vi "Pass Fail and Report Text.vi"(0 "Previous Fault Count":u8, 2 "Mode":T1, 5 "Faults Cleared":T2[](array[typedef]) {"ERD Number" format="%.0x"}, 7 "Faults Active":T2[](array[typedef]) {"ERD Number" format="%.0x"}, 9 "Motor Stopped":T2[][](array[typedef]) {"ERD Number" format="%.0x"}, 11 "Error In":errorcluster, 13 "Motor Running":T2[][](array[typedef]) {"ERD Number" format="%.0x"}) -> (4 "Pass/Fail?":bool, 6 "Report Text":string, 8 "Current Fault Count":u8, 15 "Error Out":errorcluster)   [LabVIEW 2016, in "Centauro.lvlib"]
doc: "This VI generates pass/fail and report text data based on the output of the locked rotor test VI."
uses:
  Projects/Centauro.lvlib
  Common/LabVIEW GEA2 Toolkit/LabVIEW_GEA2_Toolkit.lvlibp/type defs/ERD Read Data Out.ctl
  controls/Mode.ctl
  Common/LabVIEW GEA2 Toolkit/LabVIEW_GEA2_Toolkit.lvlibp
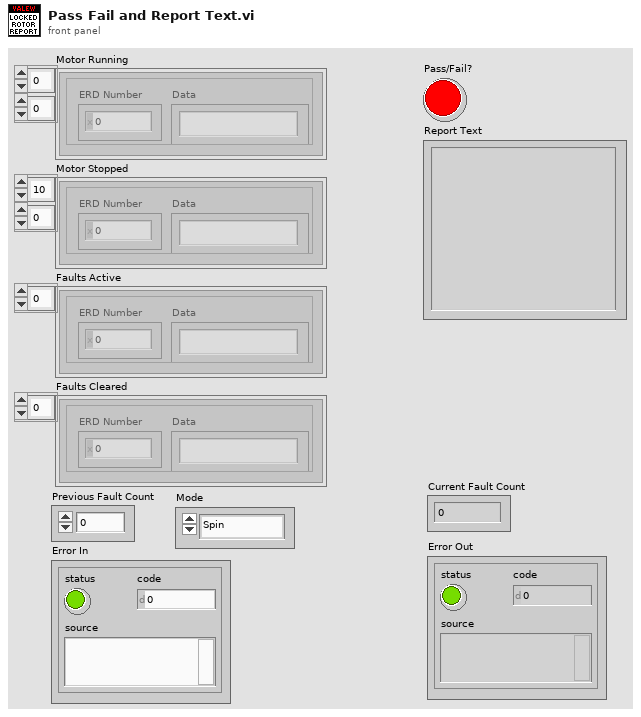
[diagram p1: front panel]
types:
  T1 = typedef "Centauro.lvlib/Mode.ctl" = enum16{"Spin", "Agitate"}
  T2 = typedef "LabVIEW_GEA2_Toolkit.lvlibp/ERD Read Data Out.ctl" = cluster{"ERD Number":u16, "Data":string}
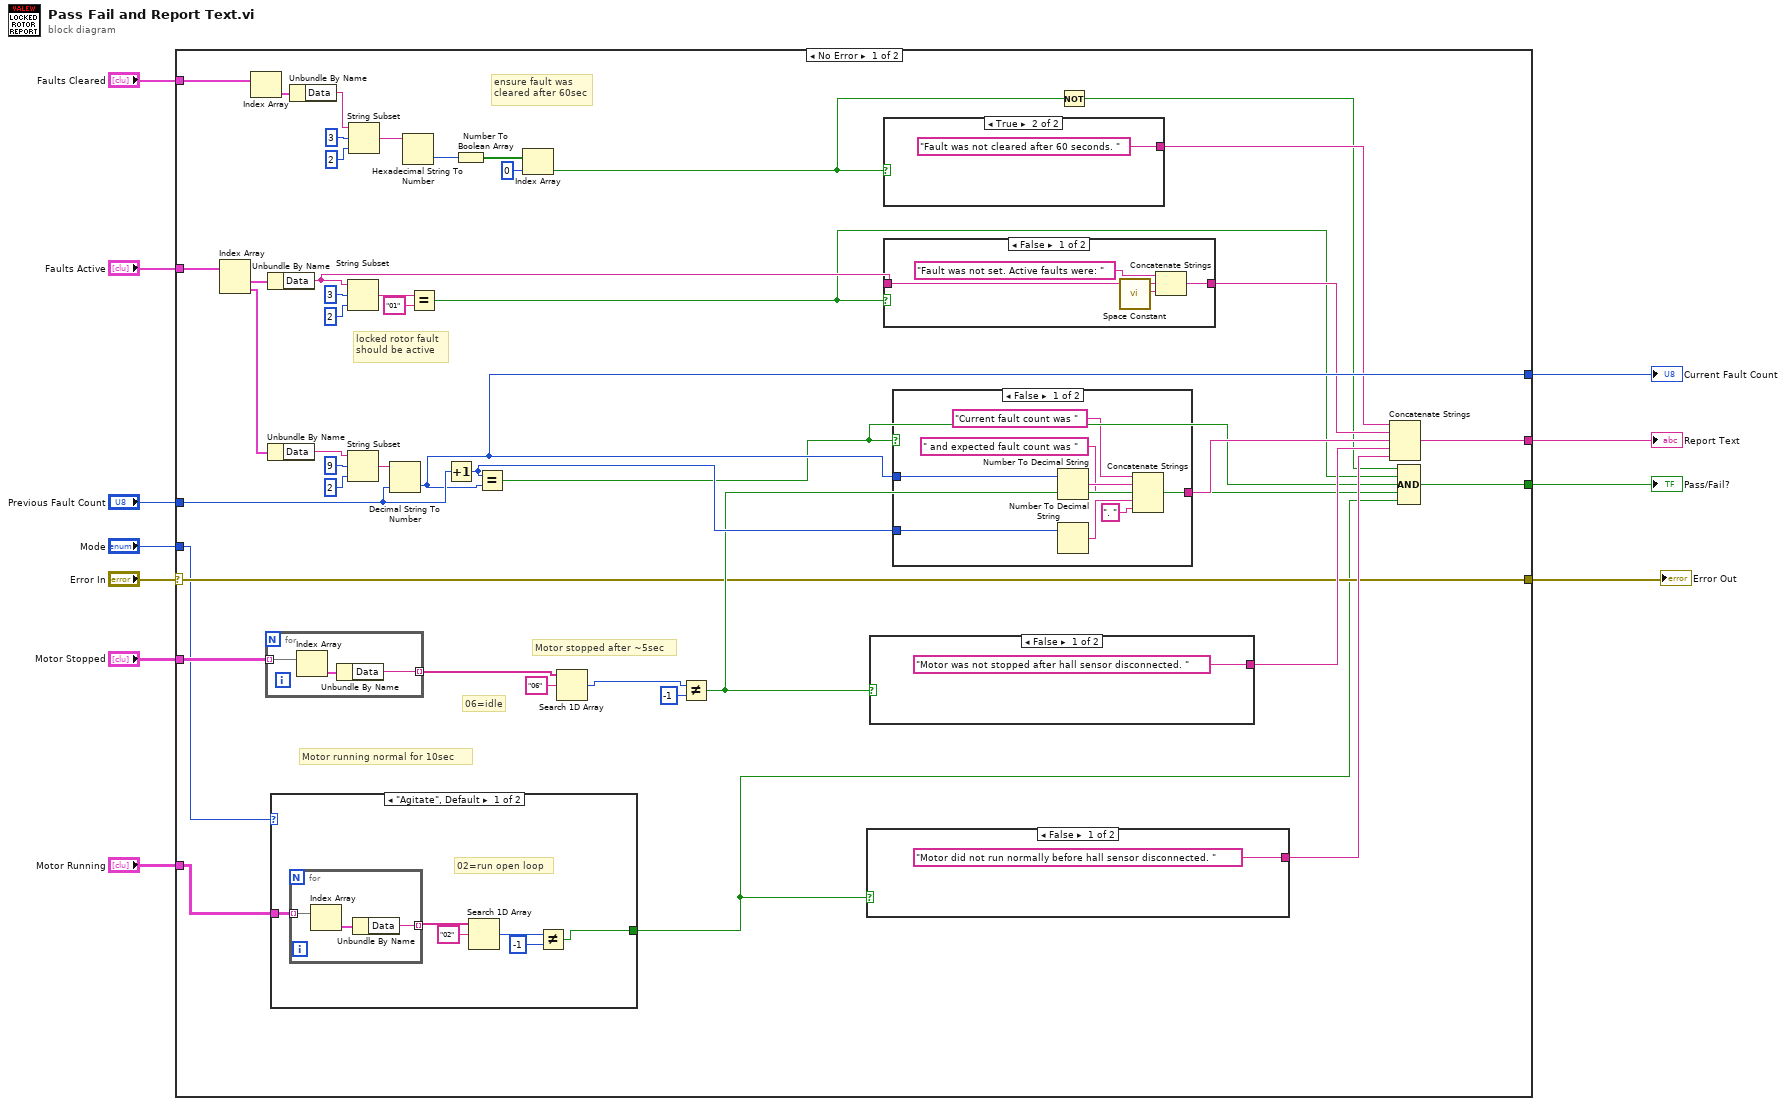
[diagram p0: block diagram]
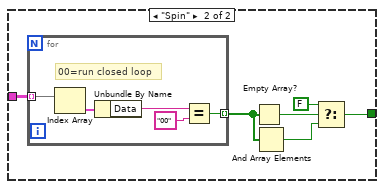
[diagram p2: hidden frame]
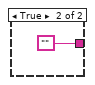
[diagram p3: hidden frame]
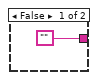
[diagram p4: hidden frame]
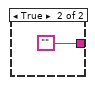
[diagram p5: hidden frame]
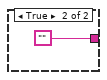
[diagram p6: hidden frame]
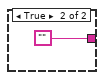
[diagram p7: hidden frame]
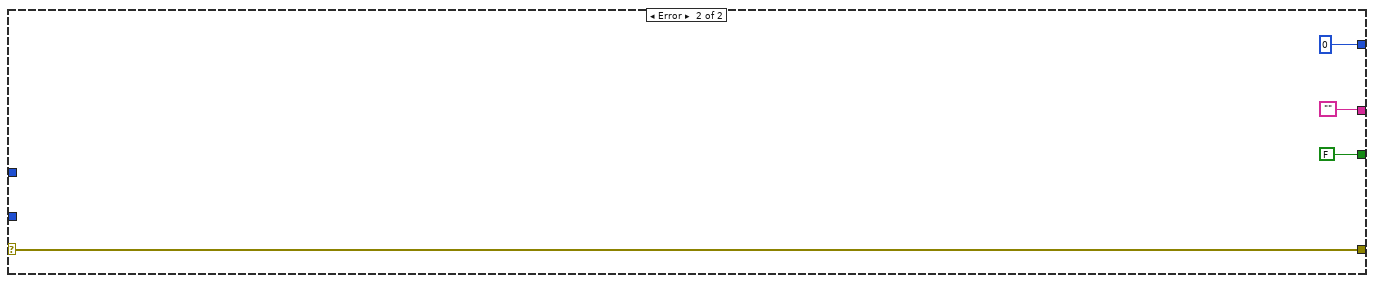
[diagram p8: hidden frame]
diagram:
  n1 = case shown="No Error" "Error In" {
    selector: "Error In" -> [w20 w103]
    tunnel: "Motor Running" -> [w56 _]
    tunnel: "Previous Fault Count" -> [w38 _]
    tunnel: "Faults Active" -> [w37 _]
    tunnel: "Faults Cleared" -> [w36 _]
    tunnel: [w34 u8 0] -> w7
    tunnel: [w27 ""] -> w6
    tunnel: [w23 FALSE] -> w5
    tunnel: "Motor Stopped" -> [w22 _]
    tunnel: [w20 w103] -> w2
    tunnel: "Mode" -> [w19 _]
    frame No Error {
      # "ensure fault was\ncleared after 60sec"
      # "locked rotor fault\nshould be active"
      # "Motor stopped after ~5sec"
      # "06=idle"
      # "Motor running normal for 10sec"
      n2 = Index Array(array=w37) -> (element #1=w52:T2, element #2=w51:T2)  [unwired: 2 in]
      n3 = Index Array(array=w36) -> (element=w50:T2)  [unwired: 1 in]
      n4 = for {
        tunnel: w22 -> [w78] mode=indexing
        tunnel: [w77] -> w21 mode=indexing
        n5 = Index Array(array=w78) -> (element=w79:T2)  [unwired: 1 in]
        n6 = Unbundle By Name(w79) -> ("Data"=w77:string)
      }
      n7 = Unbundle By Name(w52) -> ("Data"=w35:string)
      n8 = Unbundle By Name(w51) -> ("Data"=w49:string)
      n9 = case shown="\"Agitate\", Default" w19 {
        tunnel: w56 -> [w62 w71]
        tunnel: [w57 w66] -> w12
        frame "Agitate", Default {
          # "02=run open loop"
          n10 = for {
            tunnel: w62 -> [w64] mode=indexing
            tunnel: [w63] -> w61 mode=indexing
            n11 = Index Array(array=w64) -> (element=w65:T2)  [unwired: 1 in]
            n12 = Unbundle By Name(w65) -> ("Data"=w63:string)
          }
          n13 = Search 1D Array(1D array=w61, element="02") -> (index of element=w59:i32)  [unwired: 1 in]
          n14 = Not Equal?(x=w59, y=-1) -> (x != y?=w57:bool)
        }
        frame "Spin" {
          n15 = for {
            tunnel: w71 -> [w73] mode=indexing
            tunnel: [w72] -> w67 mode=indexing
            # "00=run closed loop"
            n16 = Index Array(array=w73) -> (element=w74:T2)  [unwired: 1 in]
            n17 = Unbundle By Name(w74) -> ("Data"=w75:string)
            n18 = Equal?(x=w75, y="00") -> (x = y?=w72:bool)
          }
          n19 = Empty Array?(array=w67) -> (empty?=w68:bool)
          n20 = And Array Elements(Boolean array=w67) -> (logical AND=w69:bool)
          n21 = Select(t=FALSE, s=w68, f=w69) -> (s? t:f=w66:bool)
        }
      }
      n22 = Unbundle By Name(w50) -> ("Data"=w41:string)
      n23 = String Subset(string=w35, offset (0)=3, length (rest)=2 ("length (rest)")) -> (substring=w40:string)
      n24 = String Subset(string=w49, offset (0)=9, length (rest)=2 ("length (rest)")) -> (substring=w46:string)
      n25 = String Subset(string=w41, offset (0)=3, length (rest)=2 ("length (rest)")) -> (substring=w18:string)
      n26 = Decimal String To Number(string=w46, default (0L)=w38) -> (number=w34:u8)  [unwired: 1 in, 1 out]
      n27 = Hexadecimal String To Number(string=w18) -> (number=w17:u32)  [unwired: 2 in, 1 out]
      n28 = Equal?(x=w40, y="01") -> (x = y?=w26:bool)
      n29 = Increment(x=w38) -> (x+1=w33:u8)
      n30 = Number To Boolean Array(number=w17) -> (Boolean array=w16:bool[])
      n31 = Equal?(x=w33, y=w34) -> (x = y?=w25:bool)
      n32 = Index Array(array=w16, index=0) -> (element=w14:bool)
      n33 = Search 1D Array(1D array=w21, element="06") -> (index of element=w54:i32)  [unwired: 1 in]
      n34 = Not Equal?(x=w54, y=-1) -> (x != y?=w24:bool)
      n35 = case shown="False" w12 {
        tunnel: ["Motor did not run normally before hall sensor disconnected. " ""] -> w28
        frame False {
        }
        frame True {
        }
      }
      n36 = case shown="False" w24 {
        tunnel: ["Motor was not stopped after hall sensor disconnected. " ""] -> w29
        frame False {
        }
        frame True {
        }
      }
      n37 = case shown="True" w14 {
        tunnel: ["" "Fault was not cleared after 60 seconds. "] -> w31
        frame False {
        }
        frame True {
        }
      }
      n38 = case shown="False" w26 {
        tunnel: w35 -> [w82 _]
        tunnel: [w81 ""] -> w30
        frame False {
          n39 = call <vilib>:"Space Constant.vi"() -> ("String"=w80:string)
          n40 = Concatenate Strings("Fault was not set. Active faults were: ", w82, w80) -> (w81:string)
        }
        frame True {
        }
      }
      n41 = case shown="False" w25 {
        tunnel: [w87 ""] -> w32
        tunnel: w34 -> [w93 _]
        tunnel: w33 -> [w90 _]
        frame False {
          n42 = Number To Decimal String(number=w93) -> (decimal integer string=w92:string)  [unwired: 1 in]
          n43 = Number To Decimal String(number=w90) -> (decimal integer string=w89:string)  [unwired: 1 in]
          n44 = Concatenate Strings("Current fault count was ", w92, " and expected fault count was " ("string"), w89, ". " ("string")) -> (w87:string)
        }
        frame True {
        }
      }
      n45 = Not(x=w14) -> (.not. x?=w13:bool)
      n46 = Concatenate Strings(w31, w30, w32, w29, w28) -> (w27:string)
      n47 = Compound Arithmetic op=AND(w13, w26, w25, w24, w12) -> (w23:bool)
    }
    frame Error {
    }
  }
  "Current Fault Count" <- w7
  "Report Text" <- w6
  "Pass/Fail?" <- w5
  "Error Out" <- w2
